vi "Start Logger.vi"(8 "error in (no error)":errorcluster, 11 "Worker in":refnum<class "Worker.lvclass">) -> (0 "error out":errorcluster, 2 "File Path":path, 3 "Worker out":refnum<class "Worker.lvclass">)   [LabVIEW 2016, in "Worker.lvclass"]
uses:
  Worker.lvclass
  C:/github/LabActor/Template Module/Template Module.lvclass
  Template Module/Template Module.lvclass/Template Module.ctl
  Worker.lvclass/Worker.ctl
  Loggers/Logger/Logger.lvclass/Logger.ctl
  NHMFL_Core/Libraries/File/File Class/File.lvclass/File.ctl
  Template Module/Read Logger.vi
  Read File prefix.vi
  Read Index digits.vi
  Loggers/Logger/Read File.lvclass.vi
  NHMFL_Core/Libraries/File/File Class/Write File Prefix.vi
  NHMFL_Core/Libraries/File/File Class/Write Index digits.vi
  Loggers/Logger/Write File.lvclass.vi
  Write File Path.vi
  Template Module/Write Logger.vi
  Loggers/Logger/Logger.lvclass
  NHMFL_Core/Libraries/File/File Class/File.lvclass
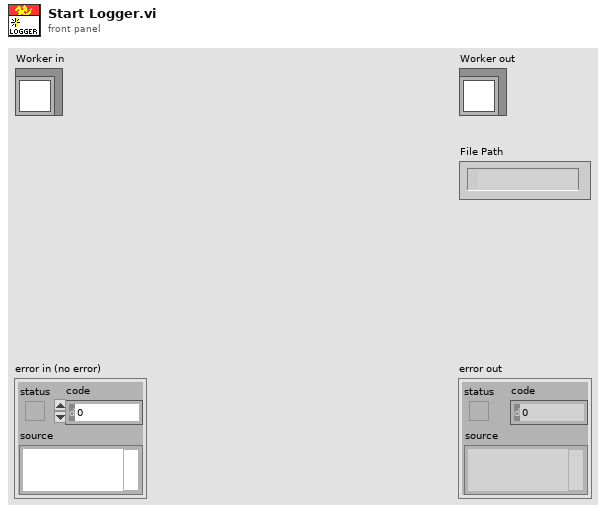
[diagram p1: front panel]
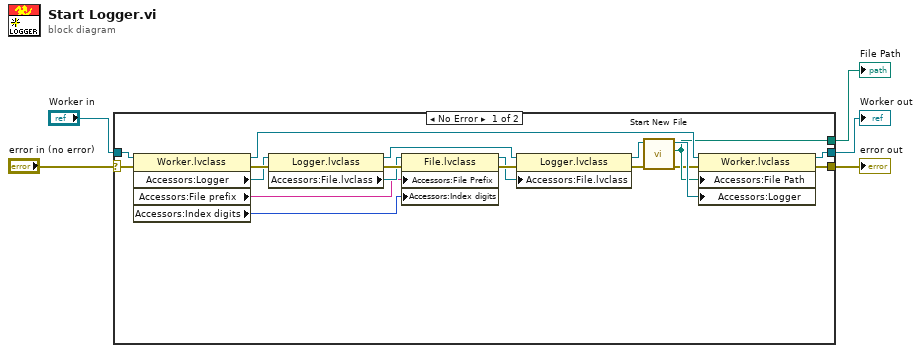
[diagram p0: block diagram]
diagram:
  n1 = case shown="No Error" "error in (no error)" {
    selector: "error in (no error)" -> [w20 w26]
    tunnel: [w22 w26] -> w4
    tunnel: [w24 w25] -> w2
    tunnel: "Worker in" -> [w23 w25]
    tunnel: [w18 _] -> w1
    frame No Error {
      n2 = property class="Worker.lvclass"(reference=w23, error in=w20) -> (reference out=w21:refnum<class "Worker.lvclass">, error out=w17:errorcluster, "Accessors:Logger"=w14:refnum<class "Logger.lvclass">, "Accessors:File prefix"=w7:string, "Accessors:Index digits"=w6:i32)
      n3 = property class="Logger.lvclass"(reference=w14, error in=w17) -> (reference out=w12:refnum<class "Logger.lvclass">, error out=w15:errorcluster, "Accessors:File.lvclass"=w9:refnum<class "File.lvclass">)
      n4 = property class="File.lvclass"(reference=w9, error in=w15, "Accessors:File Prefix"=w7, "Accessors:Index digits"=w6) -> (reference out=w8:refnum<class "File.lvclass">, error out=w10:errorcluster)
      n5 = property class="Logger.lvclass"(reference=w12, error in=w10, "Accessors:File.lvclass"=w8) -> (reference out=w11:refnum<class "Logger.lvclass">, error out=w13:errorcluster)
      n6 = call-dynamic "Start New File.vi"("error in (no error)"=w13, "Logger in"=w11) -> ("error out"=w16:errorcluster, "File Path"=w18:path, "Logger out"=w19:refnum<class "Logger.lvclass">)  [unwired: 7 in]
      n7 = property class="Worker.lvclass"(reference=w21, error in=w16, "Accessors:File Path"=w18, "Accessors:Logger"=w19) -> (reference out=w24:refnum<class "Worker.lvclass">, error out=w22:errorcluster)
    }
    frame Error {
    }
  }
  "error out" <- w4
  "Worker out" <- w2
  "File Path" <- w1
